vi "AdaptToInputs.vi"(3 "Term Types":T1[](array[typedef]), 4 "XRef":refnum<vi>, 5 "State In":T4={"Input Type"=variant(dbl 0.0), "Selection"=0, "Element Names"=[], "Type Strings"=[], "Element Types"=[]}) -> (0 "Reply":string[](array[string]), 2 "State Out":T4={"Input Type"=variant(dbl 0.0), "Selection"=0, "Element Names"=[], "Type Strings"=[], "Element Types"=[]})   [LabVIEW 2015, in "Case-Tagged-Union.xnode"]
doc: "This ability VI is called by LabVIEW during type propagation so that your XNode may adapt itself to new input types. Term Types is an array of pairs of current Term IDs and the type descriptors corresponding to them. The type descriptors are taken from the signal connected to the terminal. Unwired terminals are not included in the array. Use Reply to inform LabVIEW of any actions it needs to take.\n\nDefault behavior: None.\n\nThis ability does not provide UI and OS messages are not handled."
uses:
  Case-Tagged-Union.xnode
  State.ctl
  <vilib>/XNodeSupport/XNodeTermTypeIDPair.ctl
  <vilib>/XNodeSupport/XNodeType.ctl
  <vilib>/XNodeSupport/XNodeString.ctl
  <vilib>/regexp/Match Regular Expression.xnode
  <vilib>/Erdos Miller/LV-Scripting/LV-Scripting.lvlib
  <vilib>/Utility/Data Type/NI_Data Type.lvlib
  <vilib>/XNodeSupport/NI_XNodeSupport.lvlib
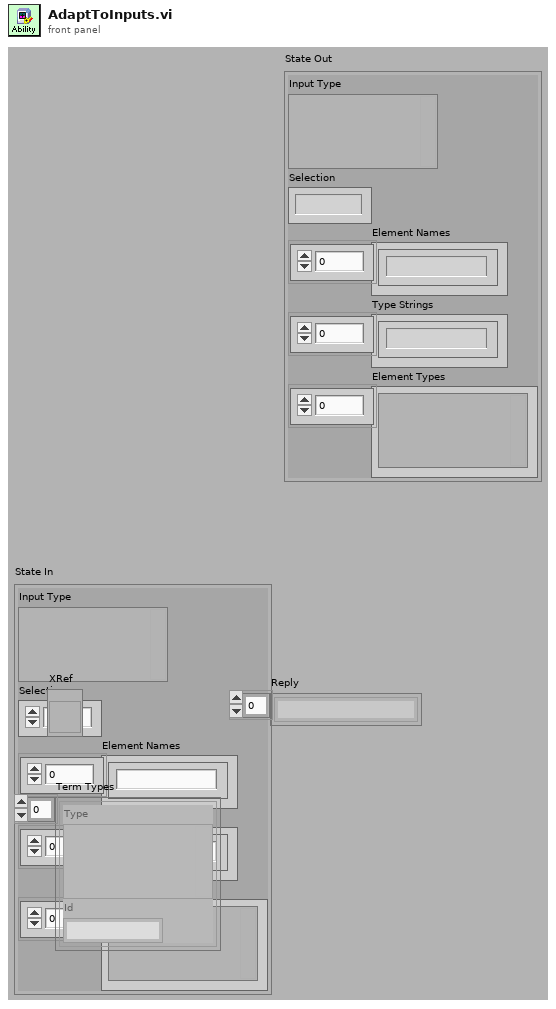
[diagram p1: front panel]
types:
  T1 = typedef "NI_XNodeSupport.lvlib/XNodeTermTypeIDPair.ctl" = cluster{"Type":T2, "Id":T3}
  T2 = typedef "NI_XNodeSupport.lvlib/XNodeType.ctl" = variant
  T3 = typedef "NI_XNodeSupport.lvlib/XNodeString.ctl" = string
  T4 = typedef "Case-Tagged-Union.xnode/State.ctl" = cluster{"Input Type":variant, "Selection":i32, "Element Names":string[], "Type Strings":string[], "Element Types":variant[]}
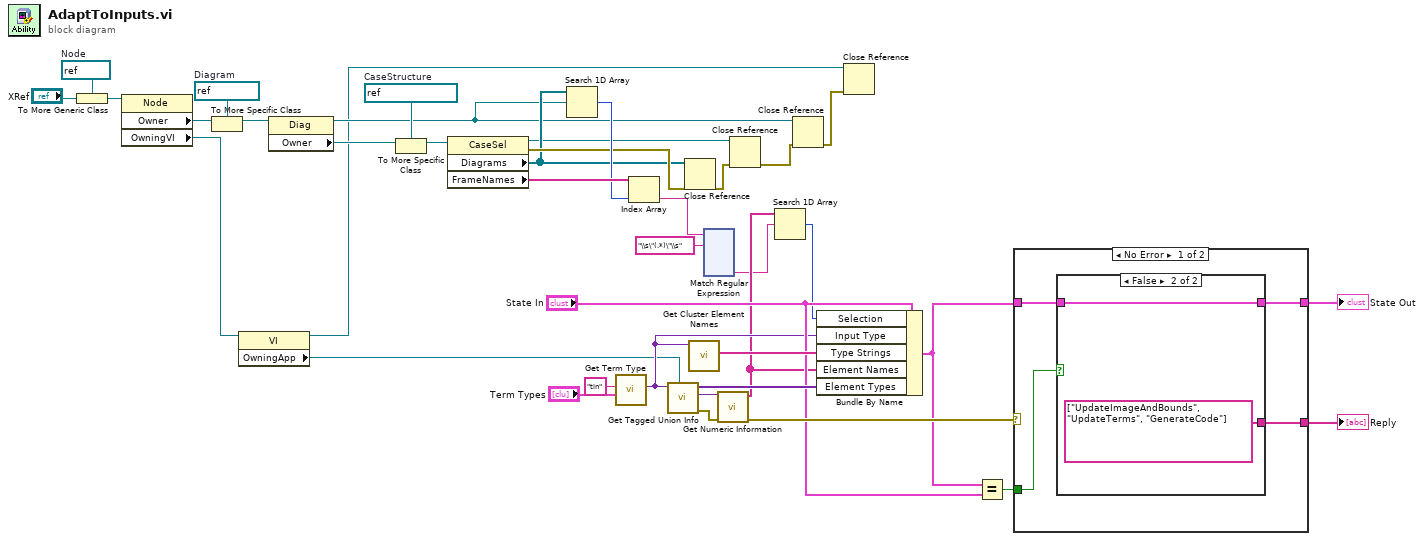
[diagram p0: block diagram]
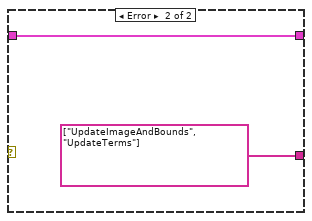
[diagram p3: hidden frame]
diagram:
  w19 = refnum<vi> refnum  # CaseStructure
  w22 = refnum<vi> refnum  # Diagram
  w25 = refnum<vi> refnum  # Node
  n1 = To More Generic Class(target class=w25, reference="XRef") -> (generic class reference=w24:refnum<vi>)
  n2 = property class="Node"(reference=w24) -> ("Owner"=w23:refnum<vi>, "OwningVI"=w3:refnum<vi>)  [unwired: 1 in, 2 out]
  n3 = To More Specific Class(target class=w22, reference=w23) -> (specific class reference=w21:refnum<vi>)  [unwired: 1 in, 1 out]
  n4 = property class="VI"(reference=w3) -> (reference out=w2:refnum<vi>, "OwningApp"=w1:refnum<vi>)  [unwired: 1 in, 1 out]
  n5 = property class="Diag"(reference=w21) -> (reference out=w6:refnum<vi>, "Owner"=w20:refnum<vi>)  [unwired: 1 in, 1 out]
  n6 = To More Specific Class(target class=w19, reference=w20) -> (specific class reference=w18:refnum<vi>)  [unwired: 1 in, 1 out]
  n7 = property class="CaseSel"(reference=w18) -> (reference out=w8:refnum<vi>, error out=w10:errorcluster, "Diagrams"=w9:refnum<vi>[], "FrameNames"=w17:string[])  [unwired: 1 in]
  n8 = Search 1D Array(1D array=w9, element=w6) -> (index of element=w16:i32)  [unwired: 1 in]
  n9 = call <vilib>:"Get Term Type.vi"("Term Types"="Term Types", "ID"="tin") -> ("Type"=w27:variant)  [unwired: 9 in]
  n10 = Index Array(array=w17, index=w16) -> (element=w12:string)
  n11 = call <vilib>:"Get Tagged Union Info.vi"("application reference (local)"=w1, "Type in"=w27) -> ("error out"=w35:errorcluster, "Enum Type"=w32:variant, "Element Types"=w31:variant[])  [unwired: 7 in]
  n12 = Close Reference(reference=w9, error in (no error)=w10) -> (error out=w7:errorcluster)
  n13 = call <vilib>:"Get Cluster Element Names.vi"("Cluster in"=w27) -> ("Names"=w34:string[])  [unwired: 8 in, 2 out]
  n14 = xnode "Match Regular Expression"("input string"=w12, "regular expression"="\\s\"(.*)\"\\s") -> ("submatch 1"=w11:string)  [unwired: 4 in, 5 out]
  n15 = call <vilib>:"Get Numeric Information.vi"("error in (no error)"=w35, "Variant"=w32) -> ("error out"=w33:errorcluster, "Enum Names"=w15:string[])  [unwired: 6 in, 2 out]
  n16 = Close Reference(reference=w8, error in (no error)=w7) -> (error out=w5:errorcluster)
  n17 = Search 1D Array(1D array=w15, element=w11) -> (index of element=w14:i32)  [unwired: 1 in]
  n18 = Close Reference(reference=w6, error in (no error)=w5) -> (error out=w4:errorcluster)
  n19 = Bundle By Name(cluster="State In", "Selection"=w14, "Input Type"=w27, "Type Strings"=w34, "Element Names"=w15, "Element Types"=w31) -> (w28:T4)
  n20 = Close Reference(reference=w2, error in (no error)=w4) -> ()  [unwired: 1 out]
  n21 = Equal?(x=w28, y="State In") -> (x = y?=w30:bool)
  n22 = case shown="No Error" w33 {
    tunnel: [w43 string[] ["UpdateImageAndBounds", "UpdateTerms"] ("Reply")] -> w37
    tunnel: w28 -> [w41 w48]
    tunnel: [w42 w48] -> w36
    tunnel: w30 -> [w40 _]
    frame No Error {
      n23 = case shown="False" w40 {
        tunnel: [_ string[] ["UpdateImageAndBounds", "UpdateTerms", "GenerateCode"] ("Reply")] -> w43
        tunnel: w41 -> [w44 w45]
        tunnel: [w44 w45] -> w42
        frame True {
        }
        frame False {
        }
      }
    }
    frame Error {
    }
  }
  "Reply" <- w37
  "State Out" <- w36
